vi "Event Notification.Initialize.vi"(4 "Parent Q":refnum<queue>, 6 "Is Child?":bool, 8 "error in (no error)":errorcluster, 9 "StatusTxtBoxRef":refnum<vi>, 10 "AppID":string, 11 "Event Notification in":refnum<class "Event Notification.lvclass">) -> (0 "error out":errorcluster, 3 "Event Notification out":refnum<class "Event Notification.lvclass">)   [LabVIEW 2024, in "EQMF.lvlib" / "Event Log.lvlib" / "Event Notification.lvclass"]
uses:
  Event Notification.lvclass
  Queues/Q.Element.ctl
  Event Notification.lvclass/Event Notification.ctl
  Queues/Queue Utils.lvlib
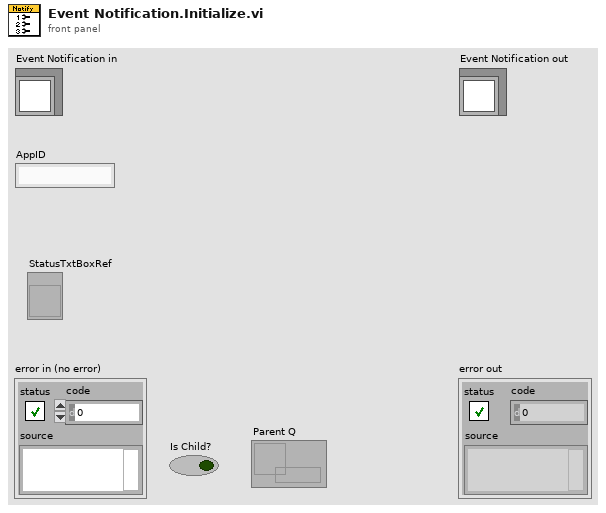
[diagram p1: front panel]
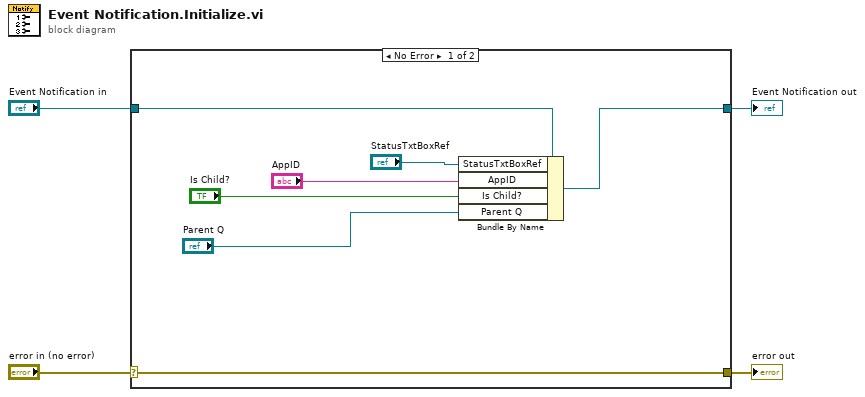
[diagram p0: block diagram]
diagram:
  n1 = case shown="No Error" "error in (no error)" {
    selector: "error in (no error)" -> [w11 w13]
    tunnel: [w11 w13] -> w3
    tunnel: [w9 w12] -> w1
    tunnel: "Event Notification in" -> [w10 w12]
    frame No Error {
      n2 = Bundle By Name(cluster=w10, "StatusTxtBoxRef"="StatusTxtBoxRef", "AppID"="AppID", "Is Child?"="Is Child?", "Parent Q"="Parent Q") -> (w9:refnum<class "Event Notification.lvclass">)
    }
    frame Error {
    }
  }
  "error out" <- w3
  "Event Notification out" <- w1
